vi "Run Bitfile2.vi"() -> ()   [LabVIEW 2011]
uses:
  <vilib>/Platform/TimedLoop/XDataNode/timing_clust.ctl
  <vilib>/Platform/TimedLoop/XDataNode/nitl_modes.ctl
  <vilib>/Platform/TimedLoop/XDataNode/wakeup.ctl
  <vilib>/FPGAPlugInAG/sbRIO-9606/niLvFpga_Open_sbRIO-9606.vi
  <vilib>/rvi/interface/common/dynamic/niFpgaDynamicAddResources.vi
  <vilib>/Utility/error.llb/Error Cluster From Error Code.vi
  <vilib>/rvi/errors/niLvFpgaAdjustHostInterfaceError.vi
  <vilib>/FPGAPlugInAG/Dynamic/niLvFpga_Close_Dynamic.vi
  <vilib>/Platform/TimedLoop/XDataNode/XDataNode.xnode
  <vilib>/rvi/interface/nirviOpenFPGA/nirviOpenFPGA.xnode
  labview/FPGA Bitfiles/natcar_FPGATarget_Top-Level_610FB000.lvbitx
  <vilib>/rvi/interface/nirviReadWriteControl/nirviReadWriteControl.xnode
  <vilib>/rvi/interface/nirviCloseFPGA/nirviCloseFPGA.xnode
  <vilib>/Platform/TimedLoop/XDataNode/XDNodeRunTimeDep.lvlib
  NiFpgaLv.dll
  <vilib>/rvi/interface/Simulation/niFpgaSimulationCallBeginRW.vi
panel:
  out "x*y":dbl
  out "x-y":dbl
  in  "Speed Kd":dbl=0.2
  out "Waveform Chart 2":dbl(graph)
  out "Waveform Chart":dbl(graph)
  out "Measured Speed [m/s]":dbl
  out "Controller Throttle":dbl
  in  "uBlaze Reset":bool
  in  "Steering ON 1e-7s":u32=15000 min=10240 max=19650 step=100
  in  "Automatic Steering":bool
  in  "Automatic Throttle":bool
  in  "GO frequency (Hz)":u16=200 min=10 max=10000 step=10
  in  "GO duty (100*%)":u16 max=100 step=1
  in  "Desired Speed [m/s]":dbl
  in  "Speed Kp":dbl=1.0
  in  "Speed Ki":dbl=0.2
  in  "STOP":bool
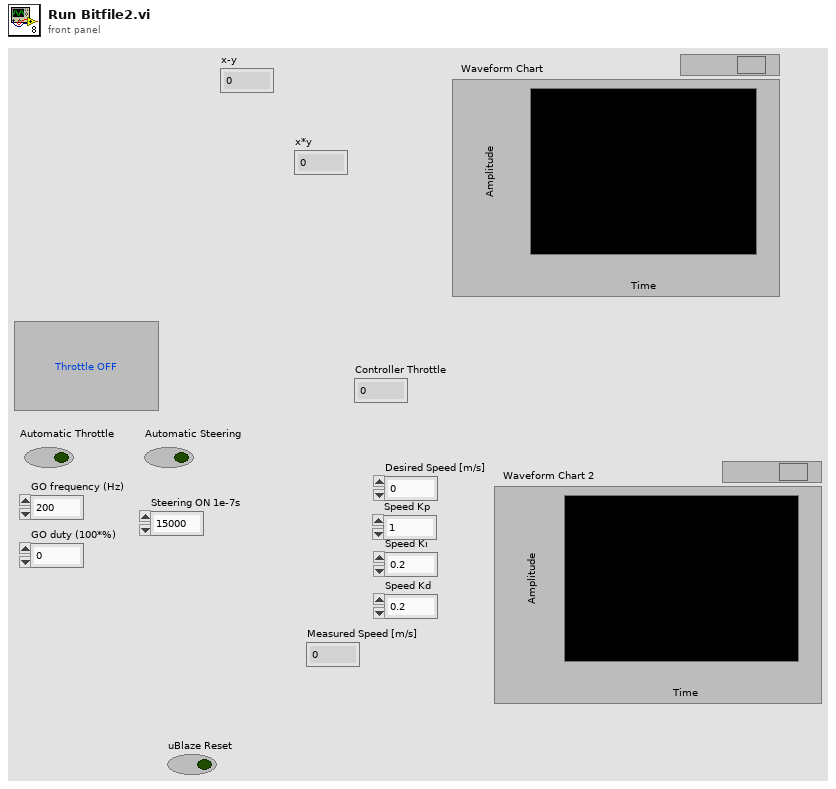
[diagram p1: front panel]
types:
  T1 = typedef "XDNodeRunTimeDep.lvlib/timing_clust.ctl" = cluster{"Expected End [f-1]":u64, "Actual End [f-1]":u64, "Finished Late? [f-1]":bool, "Expected End [i-1]":u64, "Actual End [i-1]":u64, "Finished Late? [i-1]":bool, "Expected Start [i]":u64, "Actual Start [i]":u64, "Expected Start [f]":u64, "Actual Start [f]":u64, "Source Name":string, "Structure Name":string, "Period":i64, "Deadline":i64, "Offset":i64, "Start":i64, "Priority":i32, "Timeout":i32, "Mode":T2, "Wakeup Reason":T3, "Error":errorcluster, "Source Type":string, "Secondary Source Type":string, "Global End Time":u64, "Global Start Time":u64, "Frame Duration":u64, "Iteration Duration":u64, "Assigned CPU":i32, "I/O Scan Engine Mode":u32}
  T2 = typedef "XDNodeRunTimeDep.lvlib/nitl_modes.ctl" = enum32{"No Change", "Process missed periods, maintain original phase", "Discard missed periods, maintain original phase", "Process missed periods, ignore original phase", "Discard missed periods, ignore original phase"}
  T3 = typedef "XDNodeRunTimeDep.lvlib/wakeup.ctl" = enum32{"Normal", "Aborted", "Asynchronous wakeup", "Timing source error", "Timed loop error", "Timeout"}
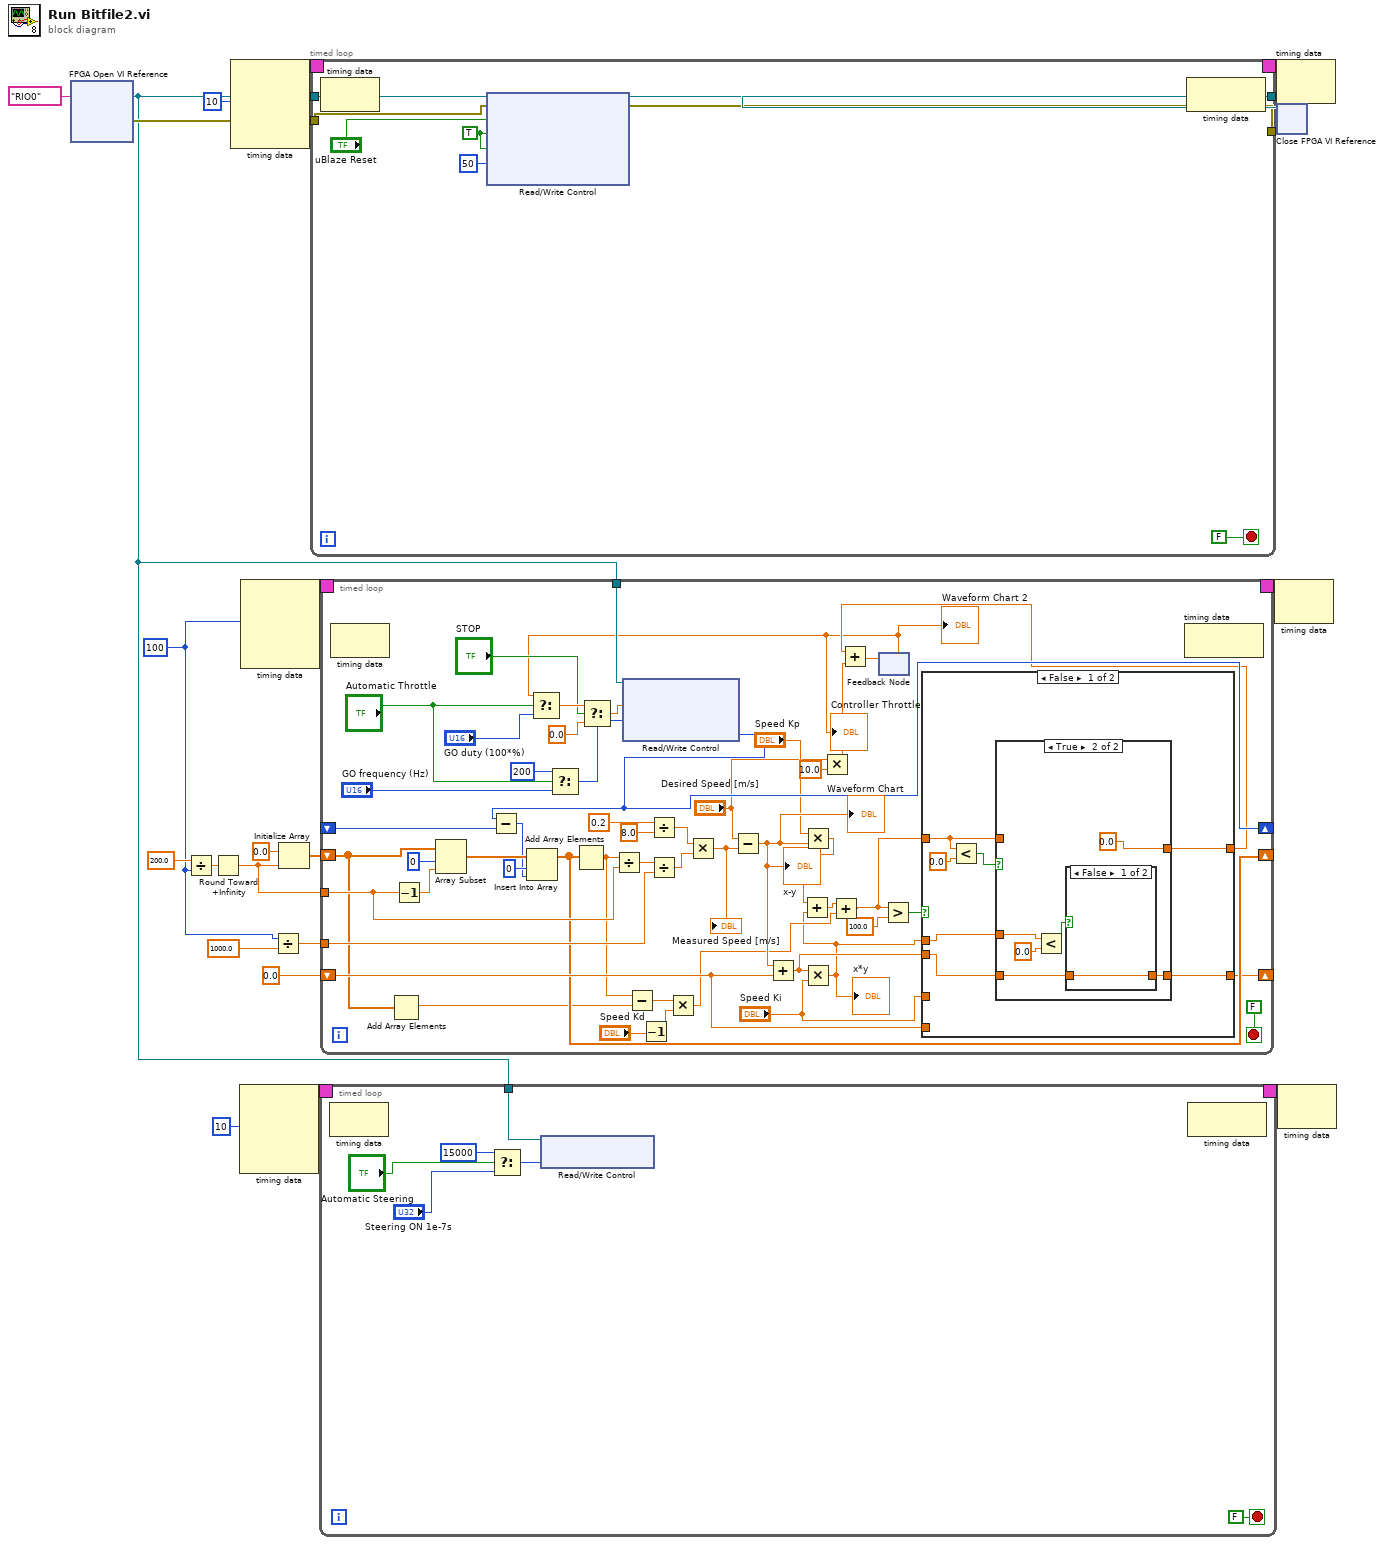
[diagram p0: block diagram]
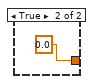
[diagram p3: hidden frame]
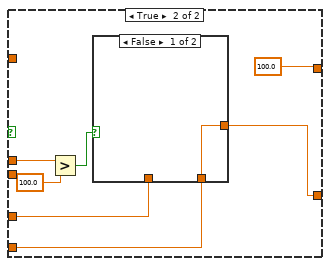
[diagram p4: hidden frame]
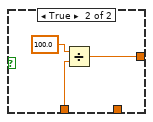
[diagram p5: hidden frame]
diagram:
  w1 = i64 100 ("Period")
  n1 = xnode "FPGA Open VI Reference"("resource name"=tag "RIO0") -> ("FPGA VI Reference Out"=w4:refnum<k20>, "error out"=w15:errorcluster)  [unwired: 1 in]
  n2 = Divide(x=200.0, y=w1) -> (x/y=w9:dbl)
  n3 = Round Toward +Infinity(x=w9) -> (ceil(x): smallest int >= x=w8:dbl)
  n4 = node-c288(i64 10 ("Period")) -> (w18:T1)  [unwired: 3 in]
  n5 = node-c288(i64 10 ("Period")) -> (w20:T1)  [unwired: 3 in]
  n6 = node-c288(w1) -> (w22:T1)  [unwired: 3 in]
  n7 = Divide(x=w1, y=1000.0) -> (x/y=w3:dbl)
  n8 = Initialize Array(0.0 ("element"), w8) -> (w12:dbl[])
  n9 = timed-loop {
    tunnel: w4 -> [w30]
    tunnel: [w29] -> w16
    tunnel: w15 -> [w27]
    tunnel: [w26] -> w14
    timing: w18 -> [_]
    timing-out: [_] -> w17
    stop <- FALSE stop-if-true
    w24 = TRUE ("manual steering")
    n10 = node-c288() -> ()  [unwired: 1 in, 1 out]
    n11 = xnode "Read/Write Control"("FPGA VI Reference In"=w30, "error in"=w27, "uBlaze Reset"="uBlaze Reset", "manual steering"=w24, "manual throttle"=w24, "Steering frequency (Hz)"=u16 50) -> ("FPGA VI Reference Out"=w29:refnum<k20>, "error out"=w26:errorcluster)  [unwired: 1 out]
    n12 = node-c288() -> ()  [unwired: 1 in, 1 out]
  }
  n13 = timed-loop {
    timing: w20 -> [_]
    timing-out: [_] -> w19
    tunnel: w4 -> [w33]
    stop <- FALSE stop-if-true
    n14 = node-c288() -> ()  [unwired: 1 in, 1 out]
    n15 = Select(t=u32 15000, s="Automatic Steering", f="Steering ON 1e-7s") -> (s? t:f=w37:u32)
    n16 = xnode "Read/Write Control"("FPGA VI Reference In"=w33, "Steering ON 1e-7s"=w37) -> ()  [unwired: 1 in, 2 out]
    n17 = node-c288() -> ()  [unwired: 1 in, 1 out]
  }
  n18 = timed-loop {
    timing: w22 -> [_]
    timing-out: [_] -> w21
    shift-right: [w74] -> _
    shift-left: w12 -> [w58]
    tunnel: w8 -> [w85]
    tunnel: w3 -> [w83]
    shift-right: [w73] -> _
    shift-left: 0.0 -> [w75]
    tunnel: w4 -> [w68]
    shift-right: [w60] -> _
    shift-left: _ -> [w63]
    stop <- FALSE stop-if-true
    n19 = node-c288() -> ()  [unwired: 1 in, 1 out]
    n20 = Add Array Elements(numeric array=w58) -> (sum=w56:dbl)
    n21 = Decrement(x=w85) -> (x-1=w87:dbl)
    n22 = Array Subset(array=w58, index=0, length=w87) -> (w64:dbl[])
    n23 = Select(t=u16 200, s="Automatic Throttle", f="GO frequency (Hz)") -> (s? t:f=w92:u16)
    n24 = Decrement(x="Speed Kd") -> (x-1=w53:dbl)
    n25 = Divide(x=0.2, y=8.0) -> (x/y=w79:dbl)
    n26 = Multiply(x="Desired Speed [m/s]", y=10.0) -> (x*y=w46:dbl)
    n27 = feedback #1() -> (w44:dbl)  [unwired: 1 in]
    "Controller Throttle" <- w44
    "Waveform Chart 2" <- w44
    n28 = Select(t=w44, s="Automatic Throttle", f="GO duty (100*%)") -> (s? t:f=w67:dbl)
    n29 = Select(t=w67, s="STOP", f=0.0 ("t")) -> (s? t:f=w70:dbl)
    n30 = xnode "Read/Write Control"("FPGA VI Reference In"=w68, "GO duty (100*%)"=w70, "GO frequency (Hz)"=w92) -> ("Velocity counts"=w60:u32)  [unwired: 1 in, 2 out]
    n31 = Subtract(x=w60, y=w63) -> (x-y=w62:u32)
    n32 = Insert Into Array(array=w64, index=0, new element=w62) -> (w74:dbl[])
    n33 = Add Array Elements(numeric array=w74) -> (sum=w57:dbl)
    n34 = Divide(x=w57, y=w85) -> (x/y=w84:dbl)
    n35 = Subtract(x=w57, y=w56) -> (x-y=w55:dbl)
    n36 = Divide(x=w84, y=w83) -> (x/y=w80:dbl)
    n37 = Multiply(x=w55, y=w53) -> (x*y=w51:dbl)
    n38 = Multiply(x=w79, y=w80) -> (x*y=w78:dbl)
    "Measured Speed [m/s]" <- w78
    n39 = Subtract(x="Desired Speed [m/s]", y=w78) -> (x-y=w59:dbl)
    "Waveform Chart" <- w59
    "x-y" <- w59
    n40 = Add(x=w59, y=w75) -> (x+y=w72:dbl)
    n41 = Multiply(x="Speed Kp", y=w59) -> (x*y=w61:dbl)
    n42 = Multiply(x=w72, y="Speed Ki") -> (x*y=w42:dbl)
    "x*y" <- w42
    n43 = Add(x=w61, y=w42) -> (x+y=w52:dbl)
    n44 = Add(x=w52, y=w51) -> (x+y=w50:dbl)
    n45 = Greater?(x=w50, y=100.0) -> (0:w76:bool)
    n46 = case shown="False" w76 {
      tunnel: w75 -> [_ w110]
      tunnel: [w98 100.0 ("y")] -> w47
      tunnel: [w97 w111] -> w73
      tunnel: w72 -> [w95 _]
      tunnel: w50 -> [w94 _]
      tunnel: w42 -> [w93 w115]
      tunnel: "Speed Ki" -> [_ w112]
      frame False {
        n47 = Less?(x=w94, y=0.0) -> (x < y?=w96:bool)
        n48 = case shown="True" w96 {
          tunnel: [w100 0.0 ("y")] -> w98
          tunnel: [w101 w103] -> w97
          tunnel: w95 -> [w101 w102]
          tunnel: w94 -> [w100 _]
          tunnel: w93 -> [_ w105]
          frame False {
          }
          frame True {
            n49 = Less?(x=w105, y=0.0) -> (x < y?=w104:bool)
            n50 = case shown="False" w104 {
              tunnel: [w108 0.0 ("y")] -> w103
              tunnel: w102 -> [w108 _]
              frame False {
              }
              frame True {
              }
            }
          }
        }
      }
      frame True {
        n51 = Greater?(x=w115, y=100.0) -> (0:w113:bool)
        n52 = case shown="False" w113 {
          tunnel: w112 -> [_ w120]
          tunnel: [w117 w118] -> w111
          tunnel: w110 -> [w117 _]
          frame False {
          }
          frame True {
            n53 = Divide(x=100.0 ("y"), y=w120) -> (x/y=w118:dbl)
          }
        }
      }
    }
    n54 = Add(x=w47, y=w46) -> (x+y=w45:dbl)
    n55 = feedback-in #1(w45) -> ()
    n56 = node-c288() -> ()  [unwired: 1 in, 1 out]
  }
  n57 = node-c288(w21) -> ()  [unwired: 1 out]
  n58 = node-c288(w17) -> ()  [unwired: 1 out]
  n59 = xnode "Close FPGA VI Reference"("FPGA VI Reference In"=w16, "error in"=w14) -> ()  [unwired: 1 out]
  n60 = node-c288(w19) -> ()  [unwired: 1 out]
